vi "Update Stack Map Color.vi"(8 "error in (no error)":errorcluster, 11 "Map Model in":refnum<class "Map Model.lvclass">) -> (0 "error out":errorcluster, 3 "Map Model out":refnum<class "Map Model.lvclass">)   [LabVIEW 2020, in "Map Model.lvlib" / "Map Model.lvclass"]
uses:
  Map Model.lvclass
  Map Model.lvclass/Map Model.ctl
  <vilib>/picture/picture.llb/Draw 4-Bit Pixmap.vi
  Stack/Stack.lvclass
panel:
  # "NOTICE -- YOU MUST LEAVE THIS NOTICE IN PLACE.\n\nCopyright (c) 2017, LIANG LIU Shawn.Liu.cn@gmail.com\nAll rights reserved.\n\nRedistribution and use in source and binary forms, with or without modification, are permitted provided that the following conditions are met:\n-Redistributions of source code must retain the above copyright notice, this list of conditions and the following disclaimer.\n-Redistributions in binary form must reproduce the above copyright notice, this list of conditions and the following disclaimer in the documentation and/or other materials provided with the distribution.\n-Neither the name of the eLp nor the names of its contributors may be used to endorse or promote products derived from this software without specific prior written permission.\n\nTHIS SOFTWARE IS PROVIDED BY THE COPYRIGHT HOLDERS AND CONTRIBUTORS \"AS IS\" AND ANY EXPRESS OR IMPLIED WARRANTIES, INCLUDING, BUT NOT LIMITED TO, THE IMPLIED WARRANTIES OF MERCHANTABILITY AND FITNESS FOR A PARTICULAR PURPOSE ARE DISCLAIMED. IN NO EVENT SHALL THE COPYRIGHT HOLDER OR CONTRIBUTORS BE LIABLE FOR ANY DIRECT, INDIRECT, INCIDENTAL, SPECIAL, EXEMPLARY, OR CONSEQUENTIAL DAMAGES (INCLUDING, BUT NOT LIMITED TO, PROCUREMENT OF SUBSTITUTE GOODS OR SERVICES; LOSS OF USE, DATA, OR PROFITS; OR BUSINESS INTERRUPTION) HOWEVER CAUSED AND ON ANY THEORY OF LIABILITY, WHETHER IN CONTRACT, STRICT LIABILITY, OR TORT (INCLUDING NEGLIGENCE OR OTHERWISE) ARISING IN ANY WAY OUT OF THE USE OF THIS SOFTWARE, EVEN IF ADVISED OF THE POSSIBILITY OF SUCH DAMAGE."
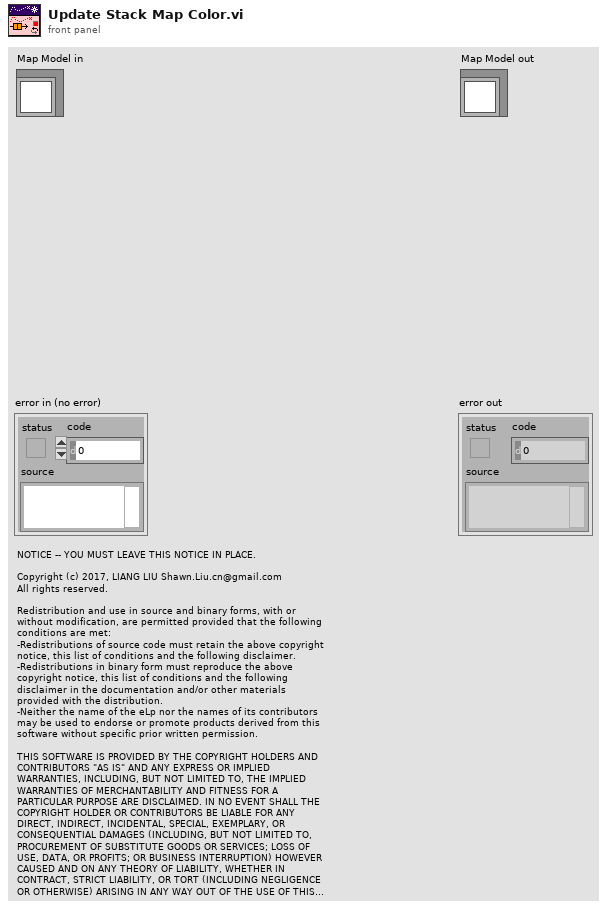
[diagram p1: front panel]
types:
  T1 = enum8{"Enabled", "Disabled", "Disabled and Grayed Out"}
  T2 = typedef "imagedata.ctl" = cluster{"image type":i32, "image depth":i32, "image":u8[], "mask":u8[], "colors":u32[], "Rectangle":cluster{"left":i16, "top":i16, "right":i16, "bottom":i16}}
  T3 = cluster{"Occupied Color":cluster{"Value":u8, "Color":u32}, "Free Color":cluster{"Value":u8, "Color":u32}, "Unknown Color":cluster{"Value":u8, "Color":u32}}
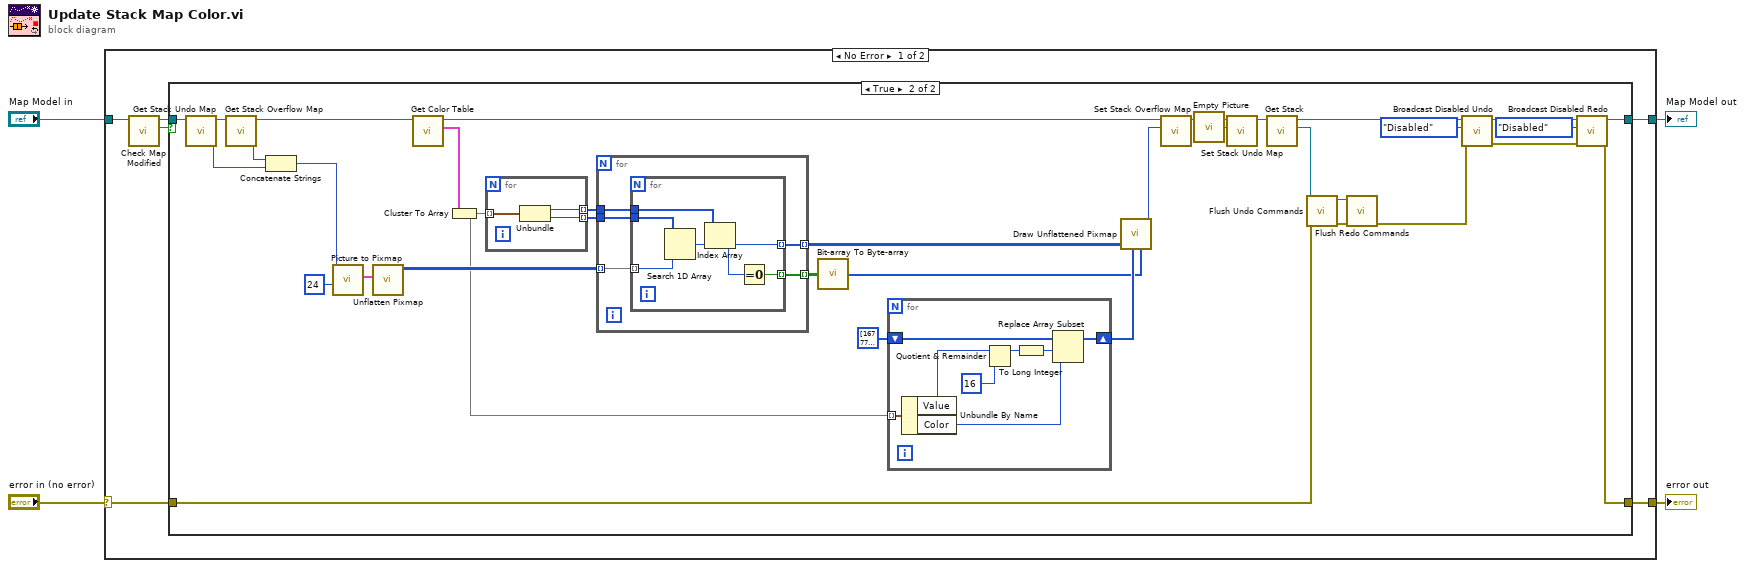
[diagram p0: block diagram]
diagram:
  n1 = case shown="No Error" "error in (no error)" {
    selector: "error in (no error)" -> [w6 w71]
    tunnel: "Map Model in" -> [w10 w70]
    tunnel: [w7 w70] -> w3
    tunnel: [w5 w71] -> w1
    frame No Error {
      n2 = call "Check Map Modified.vi"("Map Model in"=w10) -> ("Modified"=w8:bool, "Map Model out"=w9:refnum<class "Map Model.lvclass">)  [unwired: 9 in]
      n3 = case shown="True" w8 {
        tunnel: w9 -> [w12 w37]
        tunnel: [w12 w22] -> w7
        tunnel: w6 -> [w11 w16]
        tunnel: [w11 w15] -> w5
        frame False {
        }
        frame True {
          n4 = call "Get Stack Undo Map.vi"("Map Model in"=w37) -> ("Stack Undo Map"=w44:picture, "Map Model out"=w47:refnum<class "Map Model.lvclass">)  [unwired: 9 in]
          n5 = call "Get Stack Overflow Map.vi"("Map Model in"=w47) -> ("Stack Overflow Map"=w45:picture, "Map Model out"=w46:refnum<class "Map Model.lvclass">)  [unwired: 9 in]
          n6 = Concatenate Strings(w45, w44) -> (w38:picture)
          n7 = call <vilib>:"Picture to Pixmap.vi"("depth"=24, "picture"=w38) -> ("image data"=w43:T2)  [unwired: 8 in, 1 out]
          n8 = call <vilib>:"Unflatten Pixmap.vi"("image data"=w43) -> ("24-bit pixmap"=w40:u32[][])  [unwired: 4 in, 6 out]
          n9 = call "Get Color Table.vi"("Map Model in"=w46) -> ("Color Table"=w20:T3, "Map Model out"=w33:refnum<class "Map Model.lvclass">)  [unwired: 9 in]
          n10 = Cluster To Array(cluster=w20) -> (array=w21:cluster{"Value":u8, "Color":u32}[])
          n11 = for {
            tunnel: w21 -> [w58] mode=indexing
            tunnel: [w57] -> w39 mode=indexing
            tunnel: [w56] -> w41 mode=indexing
            n12 = Unbundle(w58) -> ("Value"=w57:u8, "Color"=w56:u32)
          }
          n13 = for {
            tunnel: w40 -> [w63] mode=indexing
            tunnel: [w62] -> w35 mode=indexing
            tunnel: w41 -> [w61]
            tunnel: w39 -> [w60]
            tunnel: [w59] -> w18 mode=indexing
            n14 = for {
              tunnel: w63 -> [w66] mode=indexing
              tunnel: [w65] -> w62 mode=indexing
              tunnel: w61 -> [w67]
              tunnel: w60 -> [w69]
              tunnel: [w64] -> w59 mode=indexing
              n15 = Search 1D Array(1D array=w67, element=w66) -> (index of element=w68:i32)  [unwired: 1 in]
              n16 = Index Array(array=w69, index=w68) -> (element=w65:u8)
              n17 = Equal To 0?(x=w65) -> (x = 0?=w64:bool)
            }
          }
          n18 = call <vilib>:"Bit-array To Byte-array.vi"("bit array"=w18) -> ("byte array"=w17:u8[])
          n19 = for {
            shift-right: [w54] -> w34
            shift-left: u32[] [16777215, 16776960, 128, 16711680, 16711935, 8388736, 255, 65535, 65280, 32768, 8388608, 8421376, 12632256, 8421504, 32896, 0] ("color table") -> [w55]
            tunnel: w21 -> [w53] mode=indexing
            n20 = Unbundle By Name(w53) -> ("Value"=w52:u8, "Color"=w50:u32)
            n21 = Quotient & Remainder(x=w52, y=u8 16) -> (x-y*floor(x/y)=w51:u8)  [unwired: 1 out]
            n22 = To Long Integer(number=w51) -> (32bit integer=w49:i32)
            n23 = Replace Array Subset(array=w55, new element=w50, index=w49) -> (w54:u32[])
          }
          n24 = call-poly <vilib>:"Draw Unflattened Pixmap.vi"("data"=w35, "color table"=w34, "mask"=w17) -> ("new picture"=w32:picture)  [unwired: 6 in]
          n25 = call "Set Stack Overflow Map.vi"("Stack Overflow Map"=w32, "Map Model in"=w33) -> ("Map Model out"=w23:refnum<class "Map Model.lvclass">)  [unwired: 9 in]
          n26 = call "Empty Picture"() -> ("empty picture"=w13:picture)
          n27 = call "Set Stack Undo Map.vi"("Stack Undo Map"=w13, "Map Model in"=w23) -> ("Map Model out"=w14:refnum<class "Map Model.lvclass">)  [unwired: 9 in]
          n28 = call "Get Stack.vi"("Map Model in"=w14) -> ("Stack"=w19:refnum<class "Stack.lvclass">, "Map Model out"=w26:refnum<class "Map Model.lvclass">)  [unwired: 9 in]
          n29 = call "Flush Undo Commands.vi"("error in (no error)"=w16, "Stack in"=w19) -> ("error out"=w31:errorcluster, "Stack out"=w30:refnum<class "Stack.lvclass">)  [unwired: 8 in]
          n30 = call "Flush Redo Commands.vi"("error in (no error)"=w31, "Stack in"=w30) -> ("error out"=w24:errorcluster)  [unwired: 8 in, 1 out]
          n31 = call "Broadcast Disabled Undo.vi"("error in (no error)"=w24, "Disabled Undo"=T1."Disabled", "Map Model in"=w26) -> ("error out"=w25:errorcluster, "Map Model out"=w29:refnum<class "Map Model.lvclass">)  [unwired: 7 in]
          n32 = call "Broadcast Disabled Redo.vi"("error in (no error)"=w25, "Disabled Redo"=T1."Disabled", "Map Model in"=w29) -> ("error out"=w15:errorcluster, "Map Model out"=w22:refnum<class "Map Model.lvclass">)  [unwired: 7 in]
        }
      }
    }
    frame Error {
    }
  }
  "error out" <- w1
  "Map Model out" <- w3
